vi "Initializing.vi"(10 "Timeout (ms)":i32=40000000, 11 "connection ID in":refnum<k5>) -> (2 "Timeout (ms) 2":i32, 3 "connection ID in 2":refnum<k5>)   [LabVIEW 2016]
uses:
  GrobaLimitVoltage.vi
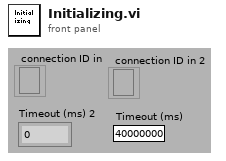
[diagram p1: front panel]
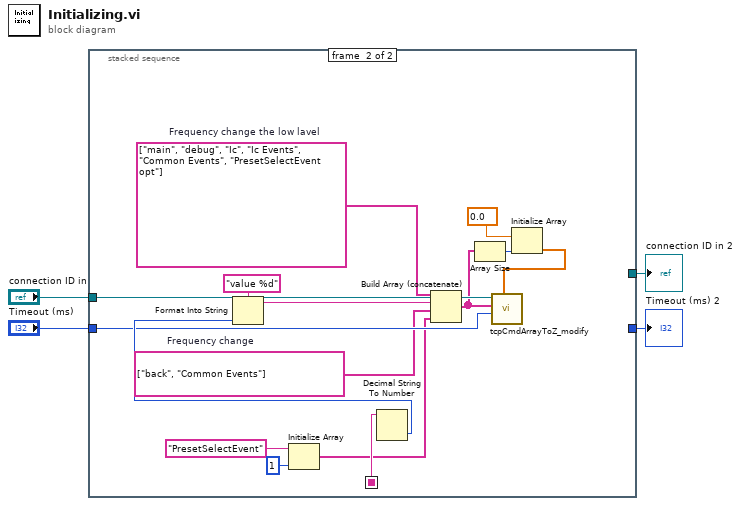
[diagram p0: block diagram]
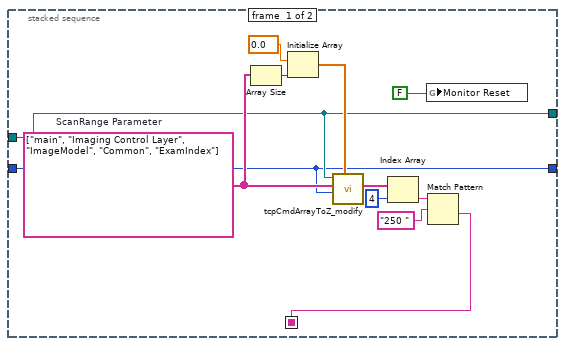
[diagram p2: hidden frame]
diagram:
  n1 = stacked-sequence {
    seq-local: [w5 _] -> [_ w22]
    tunnel: "connection ID in" -> [w7 w31]
    tunnel: "Timeout (ms)" -> [w6 w19]
    tunnel: [w7 _] -> w2
    tunnel: [w6 _] -> w1
    frame #0 {
      w16 = string[] ["main", "Imaging Control Layer", "ImageModel", "Common", "ExamIndex"]  # ScanRange Parameter
      n2 = Array Size(array=w16) -> (size(s)=w15:i32)
      n3 = Initialize Array(sgl 0.0 ("element"), w15) -> (w13:sgl[])
      n4 = call "tcpCmdArrayToZ_modify.vi"("Delay (sec)"=w13, "Timeout (ms)"=w6, "Command array"=w16, "connection ID in"=w7) -> ("Receive array"=w12:string[])  [unwired: 3 in, 4 out]
      n5 = Index Array(array=w12, index=4) -> (element=w9:string)
      n6 = global write "GrobaLimitVoltage.vi" "Monitor Reset"(FALSE) -> ()
      n7 = Match Pattern(string=w9, regular expression="250 ") -> (after substring=w5:string)  [unwired: 1 in, 3 out]
    }
    frame #1 {
      w18 = string[] ["back", "Common Events"]  # Frequency change
      w27 = string[] ["main", "debug", "Ic", "Ic Events", "Common Events", "PresetSelectEvent opt"]  # Frequency change the low lavel
      n8 = Initialize Array("PresetSelectEvent", 1 ("dimension size")) -> (w17:string[])
      n9 = Decimal String To Number(string=w22) -> (number=w21:i32)  [unwired: 2 in, 1 out]
      n10 = Format Into String(format string="value %d", w21) -> (resulting string=w26:string)  [unwired: 2 in, 1 out]
      n11 = Build Array (concatenate)(w27, w26, w18, w17) -> (w23:string[])
      n12 = Array Size(array=w23) -> (size(s)=w24:i32)
      n13 = Initialize Array(sgl 0.0 ("element"), w24) -> (w20:sgl[])
      n14 = call "tcpCmdArrayToZ_modify.vi"("Delay (sec)"=w20, "Timeout (ms)"=w19, "Command array"=w23, "connection ID in"=w31) -> ()  [unwired: 3 in, 5 out]
    }
  }
  "connection ID in 2" <- w2
  "Timeout (ms) 2" <- w1
